vi "串口助手.vi"() -> ()   [LabVIEW 2015]
doc: "实现串口通信功能，可以同时接受和发送串行数据。"
uses:
  lib/pcomm/PCOMM.lvlib
panel:
  in  "刷新按钮":bool
  out "字符串 3":string="发送控制"
  in  "DTR":bool
  in  "RTS":bool
  in  "结束位置":u32=1 max=2147483647 step=1
  in  "校验起始位":u32=1 min=1 max=2147483647 step=1
  in  "校验选项":T1(ring)
  in  "校验码":u8 format="%02x"
  in  "Open Button":bool
  in  "发送":bool
  in  "HEX发送":bool
  in  "自动发送选框":bool
  in  "自动发送时间":u32=30 caption="ms" min=1 max=2147483647 step=1
  out "字符串 2":string="接收控制"
  in  "Save Button":bool
  in  "分包显示时间":u32=30 caption="ms" min=10 step=1
  in  "HEX显示":bool
  in  "分包显示选框":bool
  in  "清空接收":bool
  in  "停止接收":bool caption="停止显示"
  out "字符串":string="串口设置"
  in  "串口号":i32(ring)=1 items=["COM1 通信端口 (COM1)"=1]
  in  "奇偶校验":i32(ring) caption="校   验" items=["None"=0, "Odd"=8, "Even"=24, "Mark"=40, "Space"=56]
  in  "数据比特":i32(ring)=3 caption="数据位" items=["5", "6", "7", "8"]
  in  "波特率":i32(ring)=16 items=["1800"=8, "2400"=9, "4800"=10, "7200"=11, "9600"=12, "19200"=13, "38400"=14, "57600"=15, "115200"=16, "230400"=17, "460800"=18, "921600"=19]
  in  "停止位":i32(ring) items=["1"=0, "2"=4]
  in  "打开/关闭串口":bool
  in  "发送文本框":string="硬石电子 携手合作,共创未来\nhttp://www.ing10bbs.com/"
  in  "自动清空数据":bool=TRUE
  in  "复位计数":bool
  in  "接收文本框":string
  out "RX":i32 min=0 step=1
  out "TX:":i32 min=0 step=1
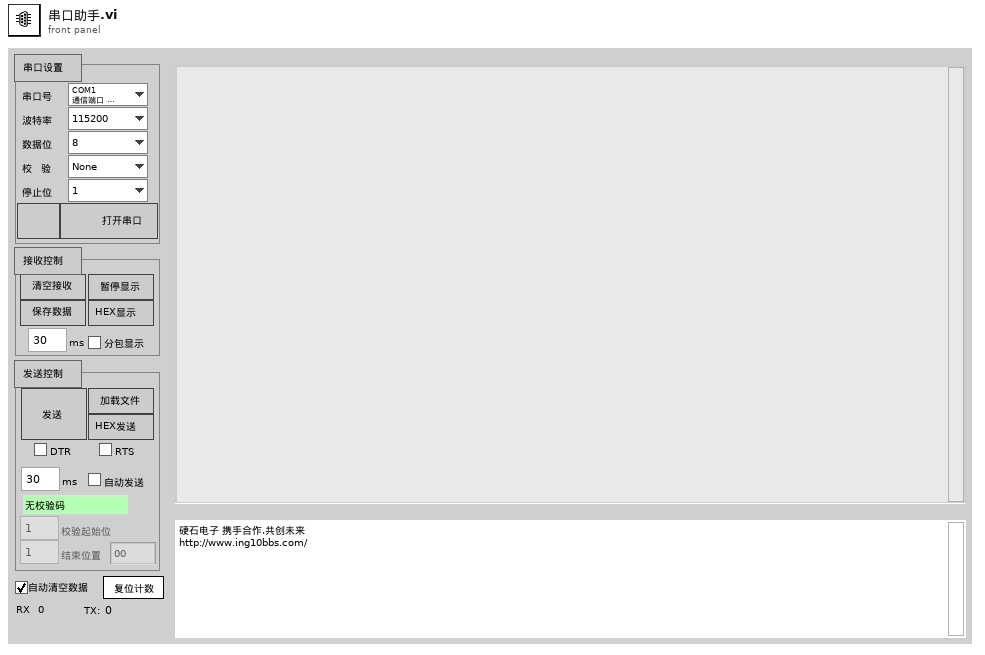
[diagram p1: front panel]
types:
  T1 = enum16{"无校验码", "校验和(0-ADD8)", "校验和(ADD8)", "异或校验(XOR8)", "固定为(BYTE)"}
  T2 = enum8{"Enabled", "Disabled", "Disabled and Grayed Out"}
  T3 = typedef "LVRectTypeDef.ctl" = cluster{"Left":i16, "Top":i16, "Right":i16, "Bottom":i16}
  T4 = typedef "LVPointTypeDef.ctl" = cluster{"Horizontal":i16, "Vertical":i16}
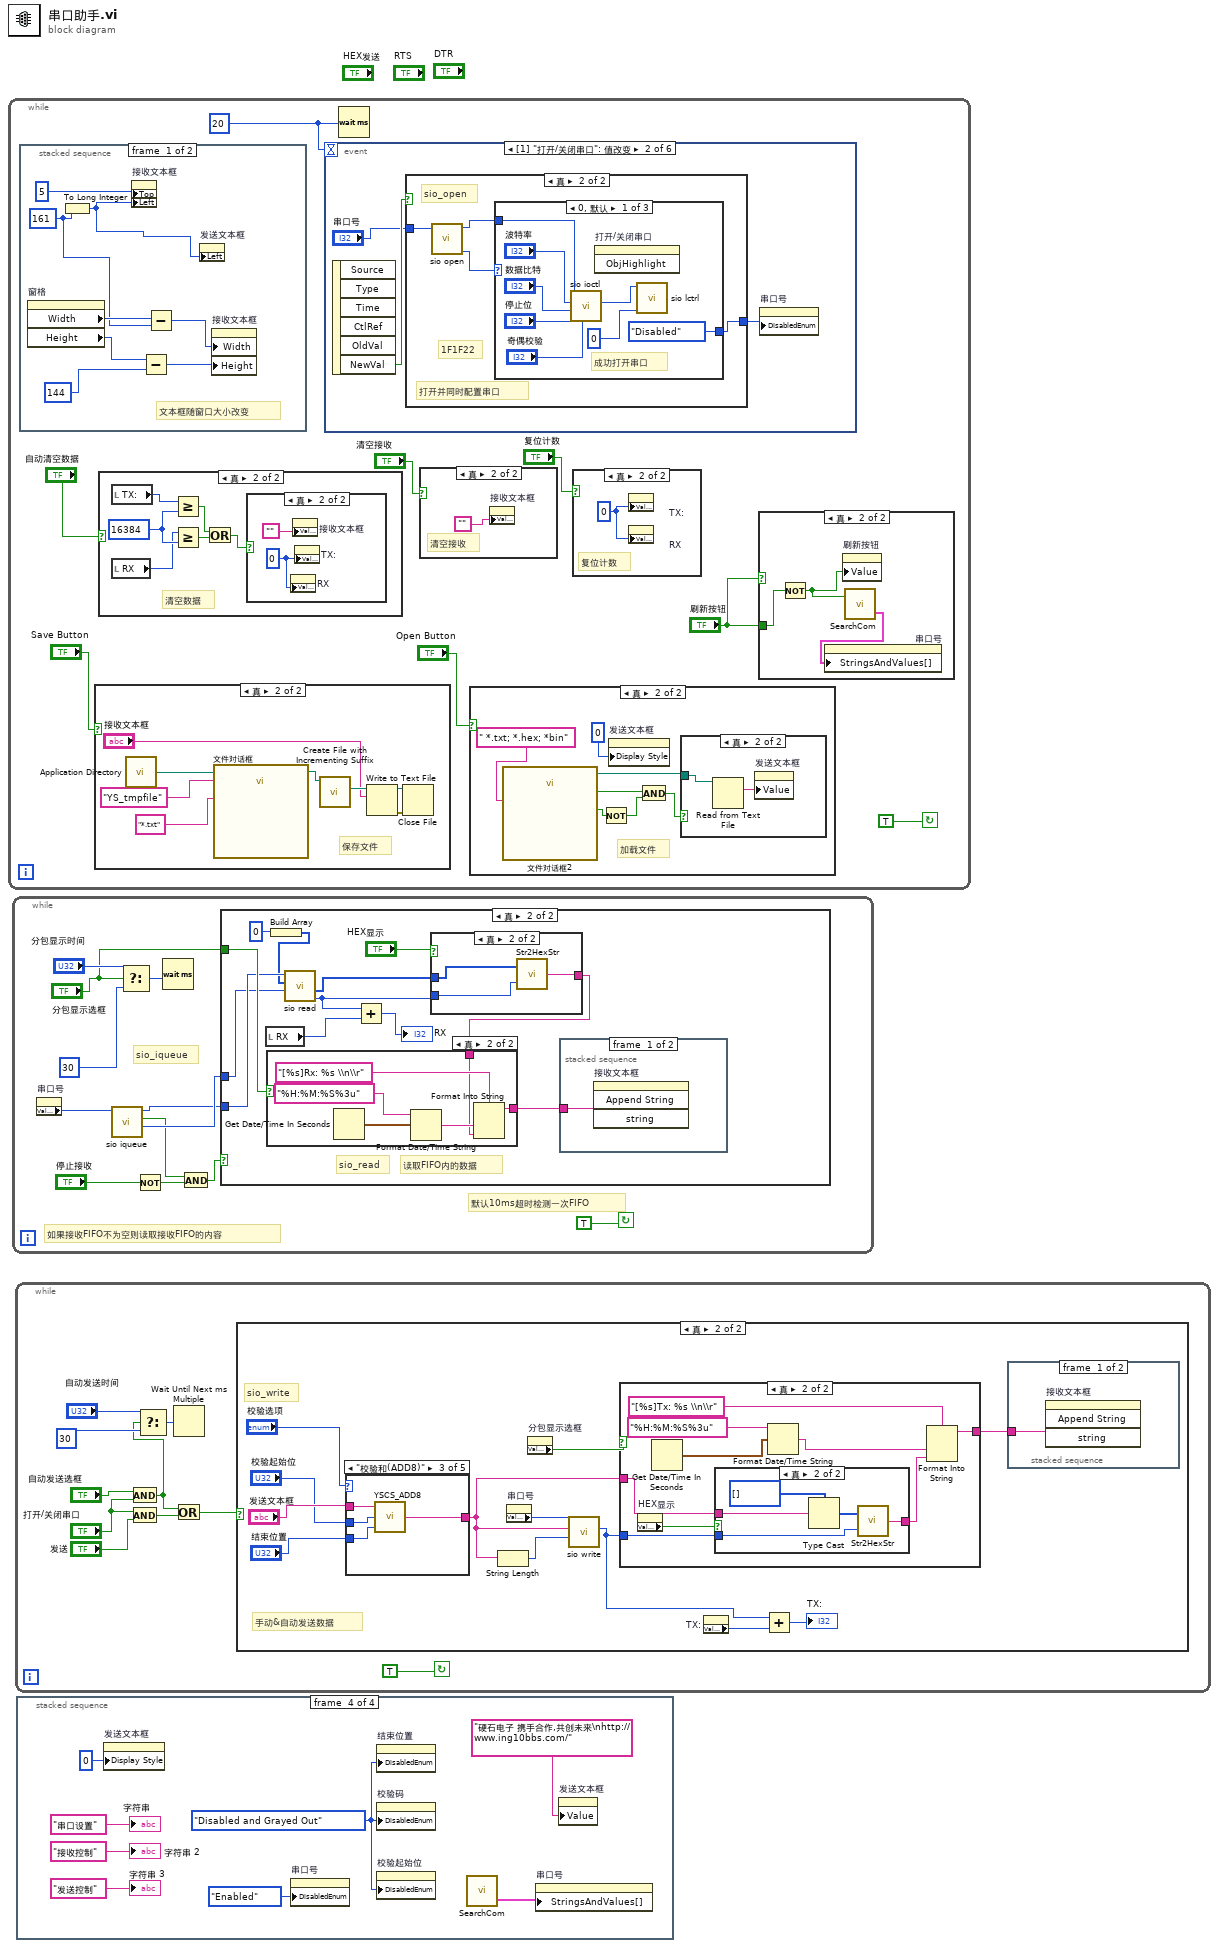
[diagram p0: block diagram]
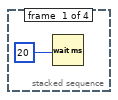
[diagram p2: hidden frame]
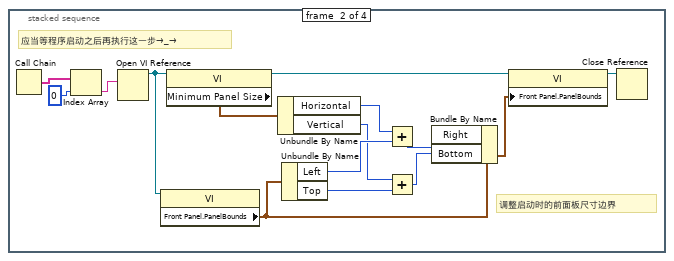
[diagram p3: hidden frame]
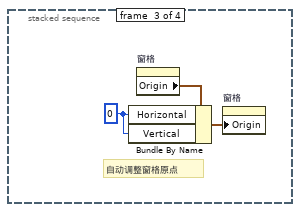
[diagram p4: hidden frame]
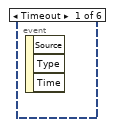
[diagram p9: hidden frame]
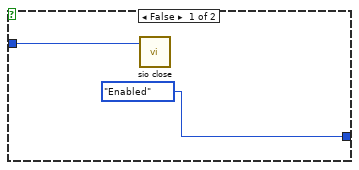
[diagram p10: hidden frame]
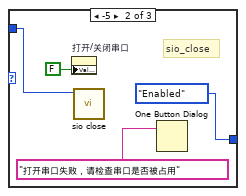
[diagram p11: hidden frame]
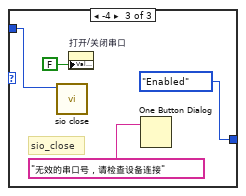
[diagram p12: hidden frame]
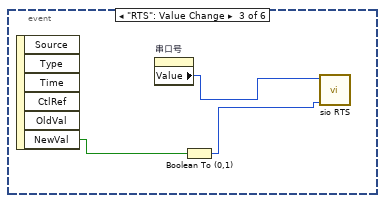
[diagram p13: hidden frame]
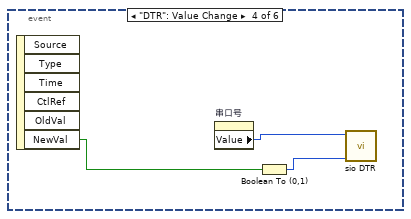
[diagram p14: hidden frame]
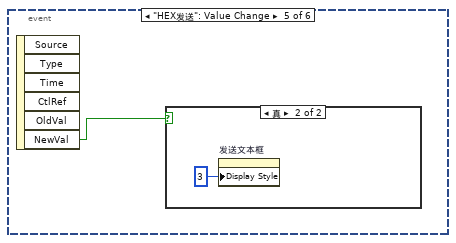
[diagram p15: hidden frame]
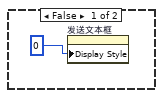
[diagram p16: hidden frame]
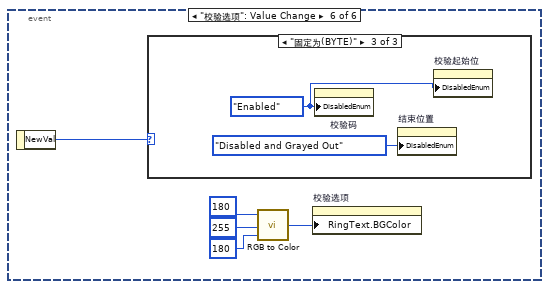
[diagram p17: hidden frame]
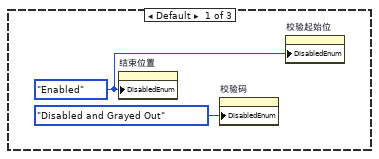
[diagram p18: hidden frame]
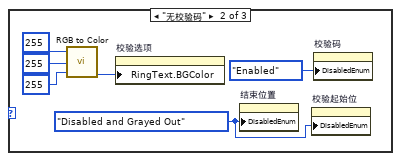
[diagram p19: hidden frame]
diagram:
  n1 = while {
    stop <- TRUE continue-if-true
    w4 = u32 20
    n2 = stacked-sequence {
      frame #0 {
        w90 = u32 161
        # "文本框随窗口大小改变"
        n3 = property on="窗格" class="Pane"() -> ("Width"=w93:u32, "Height"=w95:u32)  [unwired: 2 in, 2 out]
        n4 = To Long Integer(number=w90) -> (32bit integer=w88:i32)
        n5 = property on="接收文本框" class="Str"("Top"=5, "Left"=w88) -> ()  [unwired: 2 in, 2 out]
        n6 = Subtract(x=w95, y=u32 144) -> (x-y=w94:u32)
        n7 = Subtract(x=w93, y=w90) -> (x-y=w92:u32)
        n8 = property on="发送文本框" class="Str"("Left"=w88) -> ()  [unwired: 2 in, 2 out]
        n9 = property on="接收文本框" class="Str"("Width"=w92, "Height"=w94) -> ()  [unwired: 2 in, 2 out]
      }
      frame #1 {
        n10 = property on="接收文本框" class="Str"() -> ("Top"=w101:i32, "Height"=w102:u32, "Width"=w97:u32)  [unwired: 2 in, 2 out]
        n11 = To Unsigned Long Integer(number=w101) -> (unsigned 32bit integer=w100:u32)
        n12 = Add(x=w100, y=w102) -> (x+y=w99:u32)
        n13 = To Long Integer(number=w99) -> (32bit integer=w96:i32)
        n14 = Add(x=w96, y=27) -> ()  [unwired: 1 out]
        n15 = property on="发送文本框" class="Str"("Top"=w96, "Width"=w97) -> ()  [unwired: 2 in, 2 out]
      }
    }
    n16 = case shown="真" "Save Button" {
      frame False {
      }
      frame True {
        # "保存文件"
        n17 = call <vilib>:"Application Directory.vi"() -> ("Application Directory"=w28:path)
        n18 = call "文件对话框"("start path"=w28, "default name"="YS_tmpfile", "pattern (all files)"="*.txt") -> ("selected path"=w25:path)  [unwired: 9 in, 3 out]
        n19 = call <vilib>:"Create File with Incrementing Suffix.vi"("file path"=w25) -> ("actual path"=w22:path)  [unwired: 8 in, 2 out]
        n20 = Write to Text File(file (use dialog)=w22, text="接收文本框") -> (refnum out=w23:refnum<file>, error out=w24:errorcluster)  [unwired: 2 in, 1 out]
        n21 = Close File(refnum=w23, error in=w24) -> ()  [unwired: 2 out]
      }
    }
    n22 = case shown="真" "自动清空数据" {
      frame False {
      }
      frame True {
        w85 = 16384
        # "清空数据"
        n23 = local read "TX:"() -> (w81:i32)
        n24 = local read "RX"() -> (w80:i32)
        n25 = Greater Or Equal?(x=w81, y=w85) -> (x >= y?=w84:bool)
        n26 = Greater Or Equal?(x=w80, y=w85) -> (x >= y?=w83:bool)
        n27 = Or(x=w84, y=w83) -> (x .or. y?=w82:bool)
        n28 = case shown="真" w82 {
          frame False {
          }
          frame True {
            w86 = 0
            n29 = property on="RX" class="DigNum (严格)"("Value"=w86) -> ()  [unwired: 2 in, 2 out]
            n30 = property on="接收文本框" class="Str"("Value"="" ("空字符串常量")) -> ()  [unwired: 2 in, 2 out]
            n31 = property on="TX:" class="DigNum (严格)"("Value"=w86) -> ()  [unwired: 2 in, 2 out]
          }
        }
      }
    }
    n32 = event shown="[1] \"打开/关闭串口\": 值改变" {
      selector: _ -> [_ _ _ _ _ _]
      dyn-events: _ -> [_ _ _ _ _ _]
      timeout: w4 -> [_ _ _ _ _ _]
      event Timeout {
        n33 = event-data() -> ()  [unwired: 1 in, 3 out]
      }
      event "打开/关闭串口": Value Change {
        n34 = event-data() -> ("NewVal"=w31:bool)  [unwired: 1 in, 5 out]
        n35 = case shown="真" w31 {
          tunnel: [T2."Enabled" w37] -> w30
          tunnel: "串口号" -> [w32 w36]
          frame False {
            n36 = call "sio close.vi"("port"=w32) -> ()  [unwired: 9 in, 2 out]
          }
          frame True {
            # "1F1F22"
            # "sio_open"
            # "打开并同时配置串口"
            n37 = call "sio open.vi"("port"=w36) -> ("port"=w35:i32, "Status"=w34:i32)  [unwired: 6 in]
            n38 = case shown="0, 默认" w34 {
              tunnel: w35 -> [w44 w46 w50]
              tunnel: [T2."Disabled" T2."Enabled" T2."Enabled"] -> w37
              frame 0, Default {
                # "成功打开串口"
                n39 = call "sio ioctl.vi"("parity"="奇偶校验", "stop bits"="停止位", "data bits"="数据比特", "baud"="波特率", "port"=w44) -> ("port"=w39:i32)  [unwired: 5 in, 1 out]
                n40 = invoke on="打开/关闭串口" class="Bool (严格)" method="ObjHighlight"() -> ()  [unwired: 3 in, 3 out]
                n41 = call "sio lctrl.vi"("mode"=0, "port"=w39) -> ()  [unwired: 8 in, 2 out]
              }
              frame -5 {
                # "sio_close"
                n42 = property on="打开/关闭串口" class="Bool (严格)"("Value"=FALSE) -> ()  [unwired: 2 in, 2 out]
                n43 = call "sio close.vi"("port"=w46) -> ()  [unwired: 9 in, 2 out]
                n44 = One Button Dialog(message="打开串口失败，请检查串口是否被占用") -> ()  [unwired: 1 in, 1 out]
              }
              frame -4 {
                # "sio_close"
                n45 = call "sio close.vi"("port"=w50) -> ()  [unwired: 9 in, 2 out]
                n46 = property on="打开/关闭串口" class="Bool (严格)"("Value"=FALSE) -> ()  [unwired: 2 in, 2 out]
                n47 = One Button Dialog(message="无效的串口号，请检查设备连接") -> ()  [unwired: 1 in, 1 out]
              }
            }
          }
        }
        n48 = property on="串口号" class="Ring (严格)"("DisabledEnum"=w30) -> ()  [unwired: 2 in, 2 out]
      }
      event "RTS": Value Change {
        n49 = event-data() -> ("NewVal"=w56:bool)  [unwired: 1 in, 5 out]
        n50 = property on="串口号" class="Ring (严格)"() -> ("Value"=w55:i32)  [unwired: 2 in, 2 out]
        n51 = Boolean To (0,1)(Boolean=w56) -> (0, 1=w54:i16)
        n52 = call "sio RTS.vi"("mode"=w54, "port"=w55) -> ()  [unwired: 9 in, 1 out]
      }
      event "DTR": Value Change {
        n53 = event-data() -> ("NewVal"=w59:bool)  [unwired: 1 in, 5 out]
        n54 = property on="串口号" class="Ring (严格)"() -> ("Value"=w58:i32)  [unwired: 2 in, 2 out]
        n55 = Boolean To (0,1)(Boolean=w59) -> (0, 1=w57:i16)
        n56 = call "sio DTR.vi"("mode"=w57, "port"=w58) -> ()  [unwired: 9 in, 1 out]
      }
      event "HEX发送": Value Change {
        n57 = event-data() -> ("NewVal"=w60:bool)  [unwired: 1 in, 5 out]
        n58 = case shown="真" w60 {
          frame False {
            n59 = property on="发送文本框" class="Str"("Display Style"=u32 0) -> ()  [unwired: 2 in, 2 out]
          }
          frame True {
            n60 = property on="发送文本框" class="Str"("Display Style"=u32 3) -> ()  [unwired: 2 in, 2 out]
          }
        }
      }
      event "校验选项": Value Change {
        n61 = event-data() -> ("NewVal"=w67:T1)  [unwired: 1 in]
        n62 = case shown="\"固定为(BYTE)\"" w67 {
          frame Default {
            w68 = T2."Enabled"
            n63 = property on="结束位置" class="DigNum (严格)"("DisabledEnum"=w68) -> ()  [unwired: 2 in, 2 out]
            n64 = property on="校验码" class="DigNum (严格)"("DisabledEnum"=T2."Disabled and Grayed Out") -> ()  [unwired: 2 in, 2 out]
            n65 = property on="校验起始位" class="DigNum (严格)"("DisabledEnum"=w68) -> ()  [unwired: 2 in, 2 out]
          }
          frame "无校验码" {
            w70 = T2."Disabled and Grayed Out"
            n66 = call <vilib>:"RGB to Color.vi"("B"=u8 255, "G"=u8 255, "R"=u8 255) -> ("Color"=w75:u32)
            n67 = property on="校验选项" class="Enum (严格)"("RingText.BGColor"=w75) -> ()  [unwired: 2 in, 2 out]
            n68 = property on="结束位置" class="DigNum (严格)"("DisabledEnum"=w70) -> ()  [unwired: 2 in, 2 out]
            n69 = property on="校验起始位" class="DigNum (严格)"("DisabledEnum"=w70) -> ()  [unwired: 2 in, 2 out]
            n70 = property on="校验码" class="DigNum (严格)"("DisabledEnum"=T2."Enabled") -> ()  [unwired: 2 in, 2 out]
          }
          frame "固定为(BYTE)" {
            w76 = T2."Enabled"
            n71 = property on="校验码" class="DigNum (严格)"("DisabledEnum"=w76) -> ()  [unwired: 2 in, 2 out]
            n72 = property on="结束位置" class="DigNum (严格)"("DisabledEnum"=T2."Disabled and Grayed Out") -> ()  [unwired: 2 in, 2 out]
            n73 = property on="校验起始位" class="DigNum (严格)"("DisabledEnum"=w76) -> ()  [unwired: 2 in, 2 out]
          }
        }
        n74 = call <vilib>:"RGB to Color.vi"("B"=u8 180, "G"=u8 255, "R"=u8 180) -> ("Color"=w63:u32)
        n75 = property on="校验选项" class="Enum (严格)"("RingText.BGColor"=w63) -> ()  [unwired: 2 in, 2 out]
      }
    }
    n76 = Wait (ms)(milliseconds to wait=w4) -> ()  [unwired: 1 out]
    n77 = case shown="真" "清空接收" {
      frame False {
      }
      frame True {
        # "清空接收"
        n78 = property on="接收文本框" class="Str"("Value"="") -> ()  [unwired: 2 in, 2 out]
      }
    }
    n79 = case shown="真" "Open Button" {
      frame False {
      }
      frame True {
        # "加载文件"
        n80 = call "文件对话框2"("pattern (all files)"=" *.txt; *.hex; *bin") -> ("selected path"=w18:path, "exists"=w14:bool, "cancelled"=w17:bool)  [unwired: 11 in, 1 out]
        n81 = Not(x=w17) -> (.not. x?=w16:bool)
        n82 = property on="发送文本框" class="Str"("Display Style"=u32 0) -> ()  [unwired: 2 in, 2 out]
        n83 = And(x=w14, y=w16) -> (x .and. y?=w15:bool)
        n84 = case shown="真" w15 {
          tunnel: w18 -> [_ w19]
          frame False {
          }
          frame True {
            n85 = Read from Text File(file (use dialog)=w19) -> (text=w20:string)  [unwired: 3 in, 3 out]
            n86 = property on="发送文本框" class="Str"("Value"=w20) -> ()  [unwired: 2 in, 2 out]
          }
        }
      }
    }
    n87 = case shown="真" "复位计数" {
      frame False {
      }
      frame True {
        w79 = 0
        # "复位计数"
        n88 = property on="TX:" class="DigNum (严格)"("Value"=w79) -> ()  [unwired: 2 in, 2 out]
        n89 = property on="RX" class="DigNum (严格)"("Value"=w79) -> ()  [unwired: 2 in, 2 out]
      }
    }
    n90 = case shown="真" "刷新按钮" {
      tunnel: "刷新按钮" -> [_ w11]
      frame False {
      }
      frame True {
        n91 = Not(x=w11) -> (.not. x?=w10:bool)
        n92 = property on="刷新按钮" class="Bool (严格)"("Value"=w10) -> ()  [unwired: 2 in, 2 out]
        n93 = call "SearchCom.vi"("使用注册表？"=w10) -> ("下拉列表项"=w9:cluster{"String":string, "Value":i32}[])  [unwired: 2 in]
        n94 = property on="串口号" class="Ring (严格)"("StringsAndValues[]"=w9) -> ()  [unwired: 2 in, 2 out]
      }
    }
  }
  n95 = while {
    stop <- TRUE continue-if-true
    # "sio_iqueue"
    # "如果接收FIFO不为空则读取接收FIFO的内容"
    # "默认10ms超时检测一次FIFO"
    n96 = property on="串口号" class="Ring (严格)"() -> ("Value"=w104:i32)  [unwired: 2 in, 2 out]
    n97 = call "sio iqueue.vi"("port"=w104) -> ("len"=w106:i32, "not empty"=w103:bool, "port"=w105:i32)  [unwired: 8 in]
    n98 = Select(t="分包显示时间", s="分包显示选框", f=u32 30) -> (s? t:f=w107:u32)
    n99 = Not(x="停止接收") -> (.not. x?=w108:bool)
    n100 = Wait (ms)(milliseconds to wait=w107) -> ()  [unwired: 1 out]
    n101 = And(x=w103, y=w108) -> (x .and. y?=w109:bool)
    n102 = case shown="真" w109 {
      tunnel: w105 -> [w116 w122]
      tunnel: w106 -> [_ w121]
      tunnel: "分包显示选框" -> [_ w125]
      frame False {
        n103 = call "sio flush.vi"("func"=0, "port"=w116) -> ()  [unwired: 8 in, 2 out]
      }
      frame True {
        # "读取FIFO内的数据"
        # "sio_read"
        n104 = local read "RX"() -> (w128:i32)
        n105 = Build Array(i8 0) -> (w120:i8[])
        n106 = call "sio read.vi"("len"=w121, "buf"=w120, "port"=w122) -> ("len"=w118:i32, "buf out"=w119:i8[])  [unwired: 4 in, 2 out]
        n107 = Add(x=w118, y=w128) -> (x+y=→"RX":i32)
        n108 = case shown="真" "HEX显示" {
          tunnel: w119 -> [w139 w143]
          tunnel: w118 -> [_ w142]
          tunnel: [w140 w141] -> w123
          frame False {
            n109 = To Unsigned Byte Integer(number=w139) -> (unsigned 8bit integer=w138:u8[])
            n110 = Byte Array To String(unsigned byte array=w138) -> (string=w140:string)
          }
          frame True {
            n111 = call "Str2HexStr.vi"("数组大小"=w142, "数组"=w143) -> ("OutStr"=w141:string)
          }
        }
        n112 = case shown="真" w125 {
          tunnel: [w131 w133] -> w117
          tunnel: w123 -> [w131 w132]
          frame False {
          }
          frame True {
            n113 = Get Date/Time In Seconds() -> (seconds since 1Jan1904=w134:timestamp)
            n114 = Format Date/Time String(time format string (%c)="%H:%M:%S%3u", seconds (now)=w134) -> (date/time string=w136:string)  [unwired: 1 in]
            n115 = Format Into String(format string="[%s]Rx: %s \\n\\r", w136, w132) -> (resulting string=w133:string)  [unwired: 2 in, 1 out]
          }
        }
        n116 = stacked-sequence {
          tunnel: w117 -> [w129 _]
          frame #0 {
            n117 = invoke on="接收文本框" class="Str" method="Append String"("string"=w129) -> ()  [unwired: 3 in, 4 out]
          }
          frame #1 {
            n118 = property on="接收文本框" class="Str"("Text.Scroll Position"=u32 4294967295) -> ()  [unwired: 2 in, 2 out]
          }
        }
      }
    }
  }
  n119 = while {
    stop <- TRUE continue-if-true
    n120 = And(x="自动发送选框", y="打开/关闭串口") -> (x .and. y?=w146:bool)
    n121 = And ("与")(x="打开/关闭串口", y="发送") -> (x .and. y?=w147:bool)
    n122 = Select(t="自动发送时间", s=w146, f=u32 30) -> (s? t:f=w149:u32)
    n123 = Wait Until Next ms Multiple(millisecond multiple=w149) -> ()  [unwired: 1 out]
    n124 = Or(x=w146, y=w147) -> (x .or. y?=w145:bool)
    n125 = case shown="真" w145 {
      frame False {
      }
      frame True {
        # "sio_write"
        # "手动&自动发送数据"
        n126 = case shown="\"校验和(ADD8)\"" "校验选项" {
          tunnel: "发送文本框" -> [w184 w188 w192 w196 w200]
          tunnel: "校验起始位" -> [_ w187 w191 w195 w199]
          tunnel: "结束位置" -> [_ w186 w190 w194 _]
          tunnel: [w184 w185 w189 w193 w198] -> w154
          frame "无校验码", Default {
          }
          frame "校验和(0-ADD8)" {
            n127 = call "YSCS_0-ADD8.vi"("结束位置"=w186, "校验起始位"=w187, "输入字符串"=w188) -> ("输出字符串"=w185:string)
          }
          frame "校验和(ADD8)" {
            n128 = call "YSCS_ADD8.vi"("结束位置"=w190, "校验起始位"=w191, "输入字符串"=w192) -> ("输出字符串"=w189:string)
          }
          frame "异或校验(XOR8)" {
            n129 = call "YSCS_XOR8.vi"("结束位置"=w194, "校验起始位"=w195, "输入字符串"=w196) -> ("输出字符串"=w193:string)
          }
          frame "固定为(BYTE)" {
            n130 = call "YSCS_CB.vi"("校验码"="校验码", "校验起始位"=w199, "输入字符串"=w200) -> ("输出字符串"=w198:string)  [unwired: 1 in]
          }
        }
        n131 = String Length(string=w154) -> (length=w156:i32)
        n132 = property on="串口号" class="Ring (严格)"() -> ("Value"=w159:i32)  [unwired: 2 in, 2 out]
        n133 = property on="分包显示选框" class="Bool (严格)"() -> ("Value"=w158:bool)  [unwired: 2 in, 2 out]
        n134 = call "sio write.vi"("len"=w156, "buf"=w154, "port"=w159) -> ("Status"=w155:i32)  [unwired: 6 in, 2 out]
        n135 = case shown="真" w158 {
          tunnel: ["" w173] -> w157
          tunnel: w155 -> [_ w171]
          tunnel: w154 -> [_ w169]
          frame False {
          }
          frame True {
            n136 = property on="HEX显示" class="Bool (严格)"() -> ("Value"=w172:bool)  [unwired: 2 in, 2 out]
            n137 = Get Date/Time In Seconds() -> (seconds since 1Jan1904=w174:timestamp)
            n138 = case shown="真" w172 {
              tunnel: w171 -> [_ w183]
              tunnel: [w178 w182] -> w170
              tunnel: w169 -> [w178 w179]
              frame False {
              }
              frame True {
                n139 = Type Cast(type=u8[] [], x=w179) -> (*(type *) &x=w180:u8[])
                n140 = call "Str2HexStr.vi"("数组大小"=w183, "数组"=w180) -> ("OutStr"=w182:string)
              }
            }
            n141 = Format Date/Time String(time format string (%c)="%H:%M:%S%3u", seconds (now)=w174) -> (date/time string=w176:string)  [unwired: 1 in]
            n142 = Format Into String(format string="[%s]Tx: %s \\n\\r", w176, w170) -> (resulting string=w173:string)  [unwired: 2 in, 1 out]
          }
        }
        n143 = property on="TX:" class="DigNum (严格)"() -> ("Value"=w160:i32)  [unwired: 2 in, 2 out]
        n144 = Add(x=w155, y=w160) -> (x+y=→"TX:":i32)
        n145 = stacked-sequence {
          tunnel: w157 -> [w166 _]
          frame #0 {
            n146 = invoke on="接收文本框" class="Str" method="Append String"("string"=w166) -> ()  [unwired: 3 in, 4 out]
          }
          frame #1 {
            n147 = property on="接收文本框" class="Str"("Text.Scroll Position"=u32 4294967295) -> ()  [unwired: 2 in, 2 out]
          }
        }
      }
    }
  }
  n148 = stacked-sequence {
    frame #0 {
      n149 = Wait (ms)(milliseconds to wait=u32 20) -> ()  [unwired: 1 out]
    }
    frame #1 {
      # "调整启动时的前面板尺寸边界"
      # "应当等程序启动之后再执行这一步→_→"
      n150 = Call Chain ("调用链")() -> (call chain=w204:string[])
      n151 = Index Array(array=w204, index=0) -> (element=w202:string)
      n152 = Open VI Reference(vi path=w202) -> (vi reference=w214:refnum<vi>)  [unwired: 1 in, 5 out]
      n153 = property class="VI"(reference=w214) -> ("Front Panel.PanelBounds"=w211:T3)  [unwired: 1 in, 2 out]
      n154 = property class="VI"(reference=w214) -> (reference out=w215:refnum<vi>, "Minimum Panel Size"=w205:T4)  [unwired: 1 in, 1 out]
      n155 = Unbundle By Name(w205) -> ("Horizontal"=w212:i16, "Vertical"=w209:i16)
      n156 = Unbundle By Name(w211) -> ("Left"=w213:i16, "Top"=w208:i16)
      n157 = Add(x=w212, y=w213) -> (x+y=w210:i16)
      n158 = Add(x=w209, y=w208) -> (x+y=w207:i16)
      n159 = Bundle By Name(cluster=w211, "Right"=w210, "Bottom"=w207) -> (w206:T3)
      n160 = property class="VI"(reference=w215, "Front Panel.PanelBounds"=w206) -> (reference out=w216:refnum<vi>)  [unwired: 1 in, 1 out]
      n161 = Close Reference(reference=w216) -> ()  [unwired: 1 in, 1 out]
    }
    frame #2 {
      w219 = i16 0
      # "自动调整窗格原点"
      n162 = property on="窗格" class="Pane"() -> ("Origin"=w218:T4)  [unwired: 2 in, 2 out]
      n163 = Bundle By Name(cluster=w218, "Horizontal"=w219, "Vertical"=w219) -> (w217:T4)
      n164 = property on="窗格" class="Pane"("Origin"=w217) -> ()  [unwired: 2 in, 2 out]
    }
    frame #3 {
      w226 = T2."Disabled and Grayed Out"
      n165 = property on="发送文本框" class="Str"("Display Style"=u32 0) -> ()  [unwired: 2 in, 2 out]
      n166 = property on="串口号" class="Ring (严格)"("DisabledEnum"=T2."Enabled" ("禁用")) -> ()  [unwired: 2 in, 2 out]
      n167 = property on="结束位置" class="DigNum (严格)"("DisabledEnum"=w226) -> ()  [unwired: 2 in, 2 out]
      n168 = property on="校验码" class="DigNum (严格)"("DisabledEnum"=w226) -> ()  [unwired: 2 in, 2 out]
      n169 = property on="校验起始位" class="DigNum (严格)"("DisabledEnum"=w226) -> ()  [unwired: 2 in, 2 out]
      n170 = call "SearchCom.vi"() -> ("下拉列表项"=w221:cluster{"String":string, "Value":i32}[])  [unwired: 3 in]
      n171 = property on="串口号" class="Ring (严格)"("StringsAndValues[]"=w221) -> ()  [unwired: 2 in, 2 out]
      n172 = property on="发送文本框" class="Str"("Value"="硬石电子 携手合作,共创未来\nhttp://www.ing10bbs.com/") -> ()  [unwired: 2 in, 2 out]
      "字符串" <- "串口设置"
      "字符串 2" <- "接收控制"
      "字符串 3" <- "发送控制"
    }
  }
